vi "add_pipette_info.vi"(8 "error in (no error)":errorcluster, 10 "data array":string[](array[string]), 11 "Analysis in":refnum<class "Analysis.lvclass">) -> (0 "error out":errorcluster, 2 "data array out":string[](array[string]), 3 "Analysis out":refnum<class "Analysis.lvclass">)   [LabVIEW 2015]
doc: "input is the data array from the text file.\nThe VI searches for the pipette info and writes the data into the AnalysisObject"
uses:
  MSControl/Classes/Analysis/Analysis.lvclass
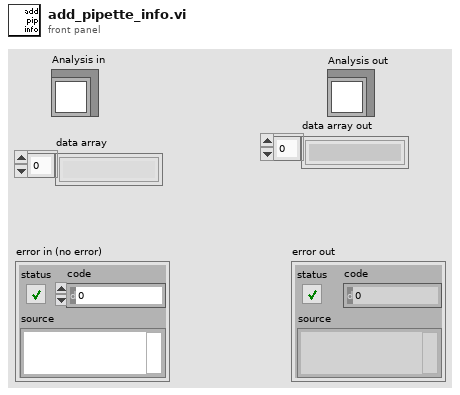
[diagram p1: front panel]
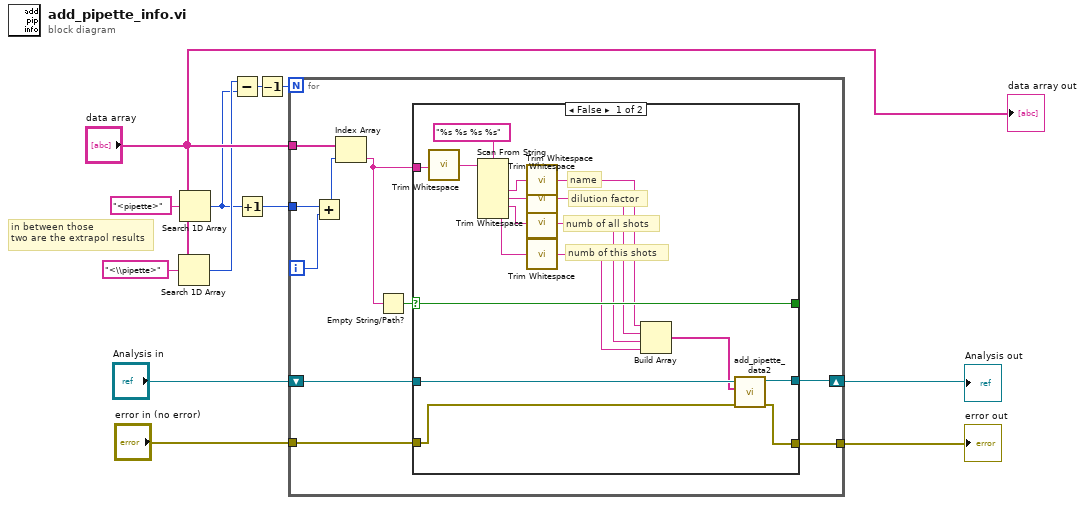
[diagram p0: block diagram]
diagram:
  # "in between those\ntwo are the extrapol results"
  n1 = Search 1D Array(1D array="data array", element="<\\pipette>") -> (index of element=w9:i32)  [unwired: 1 in]
  n2 = Search 1D Array(1D array="data array", element="<pipette>") -> (index of element=w7:i32)  [unwired: 1 in]
  n3 = Subtract(x=w9, y=w7) -> (x-y=w6:i32)
  n4 = Increment(x=w7) -> (x+1=w8:i32)
  n5 = Decrement(x=w6) -> (x-1=w5:i32)
  n6 = for {
    N: w5 -> [_]
    tunnel: "data array" -> [w22]
    tunnel: w8 -> [w21]
    tunnel: "error in (no error)" -> [w15]
    shift-right: [w14] -> w1
    shift-left: "Analysis in" -> [w16]
    tunnel: [w13] -> w2
    i -> [w20]
    n7 = Add(x=w21, y=w20) -> (x+y=w19:i32)
    n8 = Index Array(array=w22, index=w19) -> (element=w18:string)
    n9 = Empty String/Path?(string/path=w18) -> (empty?=w17:bool)
    n10 = case shown="False" w17 {
      selector: w17 -> [w36 w42]
      tunnel: w18 -> [w37 _]
      tunnel: [w36 w42] -> _
      tunnel: w16 -> [w27 w41]
      tunnel: w15 -> [w24 w40]
      tunnel: [w26 w41] -> w14
      tunnel: [w23 w40] -> w13
      frame False {
        # "numb of this shots"
        # "numb of all shots"
        # "dilution factor"
        # "name"
        n11 = call <vilib>:"Trim Whitespace.vi"("string"=w37) -> ("trimmed string"=w39:string)  [unwired: 1 in]
        n12 = Scan From String(format string="%s %s %s %s", input string=w39) -> (output 1=w35:string, output 2=w34:string, output 3=w33:string, output 4=w32:string)  [unwired: 6 in, 3 out]
        n13 = call <vilib>:"Trim Whitespace.vi"("string"=w35) -> ("trimmed string"=w31:string)  [unwired: 1 in]
        n14 = call <vilib>:"Trim Whitespace.vi"("string"=w34) -> ("trimmed string"=w30:string)  [unwired: 1 in]
        n15 = call <vilib>:"Trim Whitespace.vi"("string"=w33) -> ("trimmed string"=w29:string)  [unwired: 1 in]
        n16 = call <vilib>:"Trim Whitespace.vi"("string"=w32) -> ("trimmed string"=w28:string)  [unwired: 1 in]
        n17 = Build Array(w31, w30, w29, w28) -> (w25:string[])
        n18 = call-dynamic "add_pipette_data2.vi"("error in (no error)"=w24, "pipette data"=w25, "Analysis in"=w27) -> ("error out"=w23:errorcluster, "Analysis out"=w26:refnum<class "Analysis.lvclass">)  [unwired: 7 in]
      }
      frame True {
      }
    }
  }
  "Analysis out" <- w1
  "error out" <- w2
  "data array out" <- "data array"
